vi "GregorianCal_MonthLength.vi"(7 "Month":T1, 10 "Year (0: this year)":i32) -> (2 "Nb Days":i32)   [LabVIEW 2013]
uses:
  GregorianCal_Month -- enum.ctl
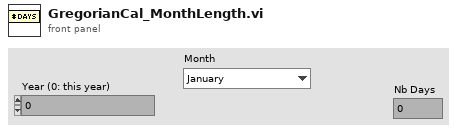
[diagram p1: front panel]
types:
  T1 = typedef "GregorianCal_Month -- enum.ctl" = enum16{"January", "February", "March", "April", "May", "June", "July", "August", "September", "October", "November", "December"}
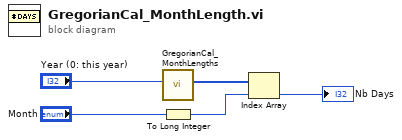
[diagram p0: block diagram]
diagram:
  n1 = call "GregorianCal_MonthLengths.vi"("Year (0: this year)"="Year (0: this year)") -> ("Month Lengths"=w4:i32[])  [unwired: 10 in]
  n2 = To Long Integer(number="Month") -> (32bit integer=w1:i32)
  n3 = Index Array(array=w4, index=w1) -> (element=→"Nb Days":i32)
